vi "terminate.vi"(8 "error in (no error)":errorcluster, 11 "GenericPlugin in":refnum<class "FPGAWrapperMH120124FrameScan_PXI7813R.lvclass">) -> (0 "error out":errorcluster, 3 "GenericPlugin out":refnum<class "FPGAWrapperMH120124FrameScan_PXI7813R.lvclass">)   [LabVIEW 2010, in "FPGAWrapperMH120124FrameScan_PXI7813R.lvclass"]
doc: "The dynamic dispatch version of this VI terminates the plug-in object by releasing all of its resources."
uses:
  FPGAWrapperMH120124FrameScan_PXI7813R.lvclass
  grabber/command_enum.ctl
  GenericFPGAWrapper/GenericFPGAWrapper/GenericFPGAWrapper.lvclass
  class_data.vi
  common/classes/ErrorController/ErrorController/class_data.vi
  common/classes/ErrorController/ErrorController/ErrorController.lvclass
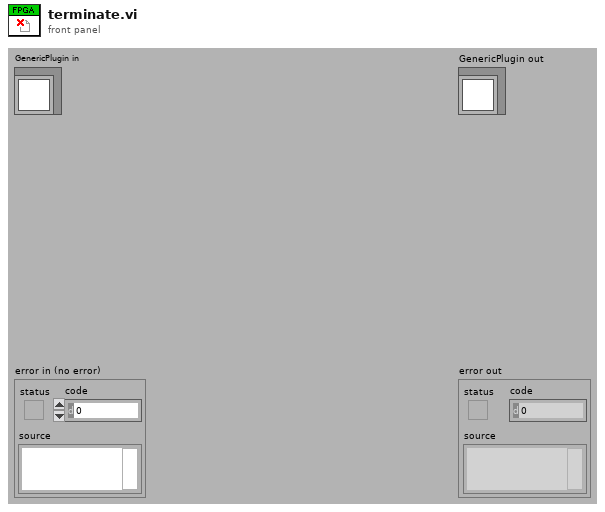
[diagram p1: front panel]
types:
  T1 = typedef "command_enum.ctl" = enum8{"NULL", "update", "start", "stop", "reset", "shut-down"}
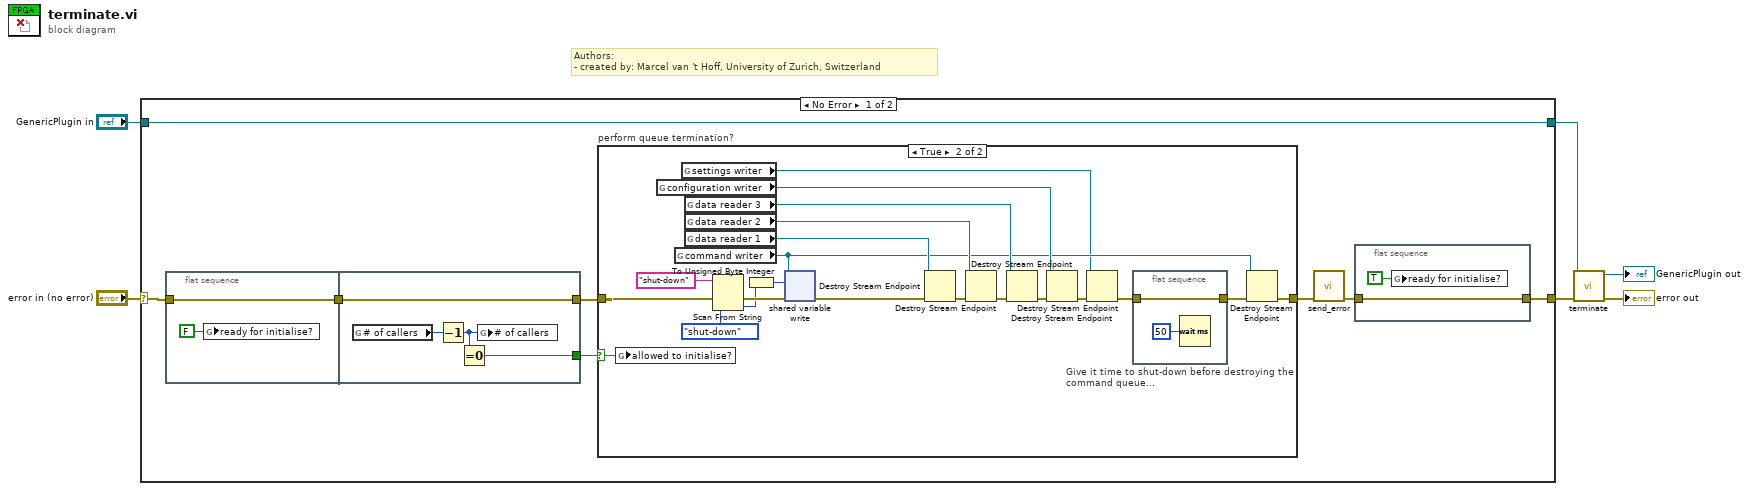
[diagram p0: block diagram]
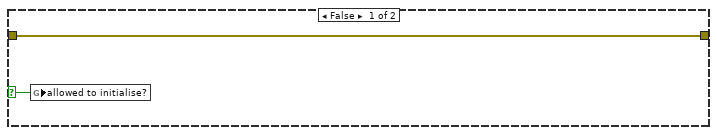
[diagram p2: hidden frame]
diagram:
  # "Authors: \n- created by: Marcel van 't Hoff, University of Zurich, Switzerland"
  n1 = case shown="No Error" "error in (no error)" {
    selector: "error in (no error)" -> [w10 w48]
    tunnel: "GenericPlugin in" -> [w14 w49]
    tunnel: [w14 w49] -> w1
    tunnel: [w11 w48] -> w3
    frame No Error {
      n2 = flat-sequence {
        tunnel: w10 -> [w16]
        tunnel: [w16] -> w8
        tunnel: [w20] -> w9
        tunnel: w8 -> [w20]
        tunnel: [w17] -> w7
        frame #0 {
          n3 = global write "class_data.vi" "ready for initialise?"(FALSE ("ready for initialise?")) -> ()
        }
        frame #1 {
          n4 = global read "class_data.vi" "# of callers"() -> (w18:i32)
          n5 = Decrement(x=w18) -> (x-1=w19:i32)
          n6 = Equal To 0?(x=w19) -> (x = 0?=w17:bool)
          n7 = global write "class_data.vi" "# of callers"(w19) -> ()
        }
      }
      n8 = case "perform queue termination?" shown="True" w7 {
        selector: w7 -> [w23 w26]
        tunnel: w9 -> [w24 w31]
        tunnel: [w24 w35] -> w13
        frame False {
          n9 = global write "class_data.vi" "allowed to initialise?"(w23) -> ()
        }
        frame True {
          n10 = global write "class_data.vi" "allowed to initialise?"(w26) -> ()
          n11 = global read "class_data.vi" "configuration writer"() -> (w38:refnum<k21>)
          n12 = global read "class_data.vi" "command writer"() -> (w37:refnum<k21>)
          n13 = global read "class_data.vi" "settings writer"() -> (w32:refnum<k21>)
          n14 = global read "class_data.vi" "data reader 3"() -> (w39:refnum<k21>)
          n15 = global read "class_data.vi" "data reader 2"() -> (w40:refnum<k21>)
          n16 = global read "class_data.vi" "data reader 1"() -> (w41:refnum<k21>)
          n17 = Scan From String(input string="shut-down", error in=w31, default 1=command_enum."shut-down" ("command")) -> (error out=w30:errorcluster, output 1=w28:T1)  [unwired: 2 in, 2 out]
          n18 = To Unsigned Byte Integer(number=w28) -> (unsigned 8bit integer=w45:u8)
          n19 = shared-variable-write(w37, w30, w45) -> (w25:errorcluster)  [unwired: 1 in, 2 out]
          n20 = Destroy Stream Endpoint(8:w25, 11:w41) -> (0:w44:errorcluster)
          n21 = Destroy Stream Endpoint(8:w44, 11:w40) -> (0:w43:errorcluster)
          n22 = Destroy Stream Endpoint(8:w43, 11:w39) -> (0:w42:errorcluster)
          n23 = Destroy Stream Endpoint(8:w42, 11:w38) -> (0:w34:errorcluster)
          n24 = Destroy Stream Endpoint(8:w34, 11:w32) -> (0:w33:errorcluster)
          n25 = flat-sequence "Give it time to shut-down before destroying the command queue..." {
            tunnel: [w46] -> w36
            tunnel: w33 -> [w46]
            frame #0 {
              n26 = Wait (ms)(milliseconds to wait=u32 50) -> ()  [unwired: 1 out]
            }
          }
          n27 = Destroy Stream Endpoint(8:w36, 11:w37) -> (0:w35:errorcluster)
        }
      }
      n28 = call "send_error.vi"("error in (no error)"=w13) -> ("error out"=w12:errorcluster)  [unwired: 10 in]
      n29 = flat-sequence {
        tunnel: [w22] -> w11
        tunnel: w12 -> [w22]
        frame #0 {
          n30 = global write "class_data.vi" "ready for initialise?"(TRUE ("ready for initialise?")) -> ()
        }
      }
    }
    frame Error {
    }
  }
  n31 = call-parent "terminate.vi"("error in (no error)"=w3, "GenericPlugin in"=w1) -> ("error out"=→"error out":errorcluster, "GenericPlugin out"=→"GenericPlugin out":refnum<class "FPGAWrapperMH120124FrameScan_PXI7813R.lvclass">)  [unwired: 8 in]
